vi "Write fcenter.vi"(8 "error in (no error)":errorcluster, 10 "fcenter":i16, 11 "Update Chirp CMD in":refnum<class "Update Chirp CMD.lvclass">) -> (0 "error out":errorcluster, 3 "Update Chirp CMD out":refnum<class "Update Chirp CMD.lvclass">)   [LabVIEW 2017, in "gPAS Library.lvlib" / "Update Chirp CMD.lvclass"]
uses:
  Update Chirp CMD.lvclass
  Update Chirp CMD.lvclass/Update Chirp CMD.ctl
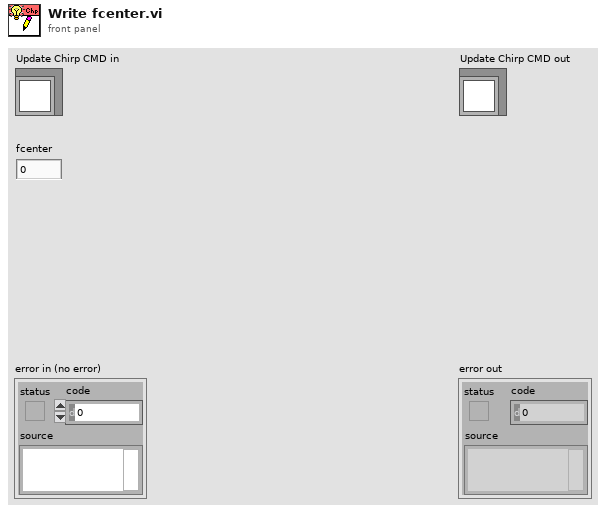
[diagram p1: front panel]
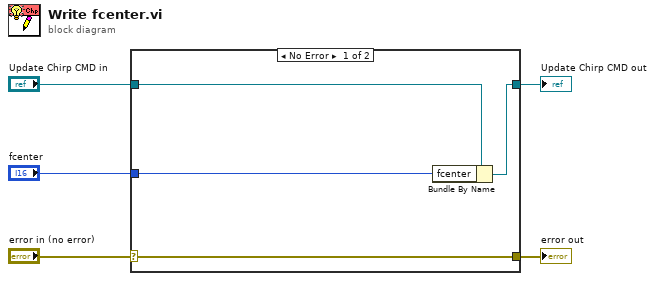
[diagram p0: block diagram]
diagram:
  n1 = case shown="No Error" "error in (no error)" {
    selector: "error in (no error)" -> [w9 w10]
    tunnel: [w9 w10] -> w4
    tunnel: [w7 w11] -> w2
    tunnel: "Update Chirp CMD in" -> [w8 w11]
    tunnel: "fcenter" -> [w6 _]
    frame No Error {
      n2 = Bundle By Name(cluster=w8, "fcenter"=w6) -> (w7:refnum<class "Update Chirp CMD.lvclass">)
    }
    frame Error {
    }
  }
  "error out" <- w4
  "Update Chirp CMD out" <- w2
